vi "Get Data Replay Loop Component Properties.vi"(8 "error in (no error)":errorcluster, 11 "Item Ref in":T3 format="%.0x") -> (0 "error out":errorcluster, 2 "DataReplayLoops":T1[](array[typedef]), 3 "Item Ref out":T3 format="%.0x")   [LabVIEW 2011, in "Engine Sim System Explorer.lvlib"]
uses:
  Engine Sim System Explorer.lvlib
  <vilib>/NI Veristand/Custom Device API/Custom Device Item Ref.ctl
  TypeDefs/DataReplayLoopComp.ctl
  TypeDefs/DataReplayComp.ctl
  Shared/Engine Simulation Global.vi
  <vilib>/NI Veristand/Custom Device API/Get Item Property (I32).vi
  <vilib>/NI Veristand/Custom Device API/Get Item Property (String).vi
  Engine Simulation Shared.lvlib
  <vilib>/NI Veristand/Custom Device API/Custom Device API.lvlib
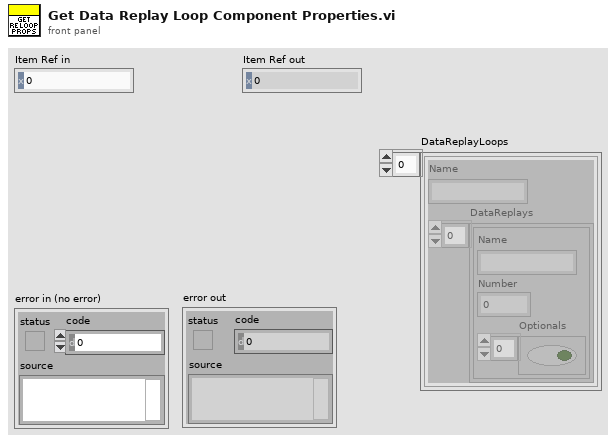
[diagram p1: front panel]
types:
  T1 = typedef "Engine Sim System Explorer.lvlib/DataReplayLoopComp.ctl" = cluster{"Name":string, "DataReplays":T2[]}
  T2 = typedef "Engine Sim System Explorer.lvlib/DataReplayComp.ctl" = cluster{"Name":string, "Number":i32, "Optionals":bool[]}
  T3 = typedef "Custom Device API.lvlib/Custom Device Item Ref.ctl" = u64
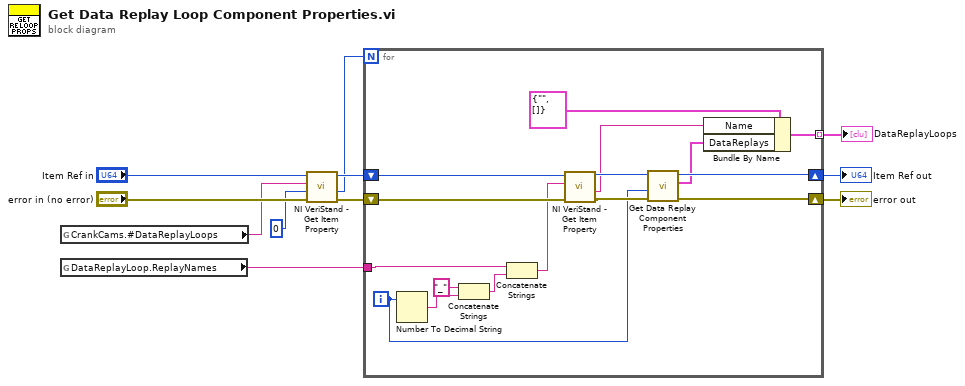
[diagram p0: block diagram]
diagram:
  n1 = global read "Engine Simulation Global.vi" "CrankCams.#DataReplayLoops"() -> (w9:string)
  n2 = global read "Engine Simulation Global.vi" "DataReplayLoop.ReplayNames"() -> (w6:string)
  n3 = call-poly <vilib>:"NI VeriStand - Get Item Property.vi"("error in (no error)"="error in (no error)", "Default Value"=0, "Property Name"=w9, "Item Ref in"="Item Ref in") -> ("error out"=w8:errorcluster, "Value"=w2:i32, "Item Ref out"=w7:T3)  [unwired: 4 in, 1 out]
  n4 = for {
    N: w2 -> [_]
    shift-right: [w17] -> w5
    shift-left: w8 -> [w24]
    shift-right: [w18] -> w4
    shift-left: w7 -> [w23]
    tunnel: w6 -> [w27]
    tunnel: [w12] -> w1 mode=indexing
    i -> [w16]
    n5 = Number To Decimal String(number=w16) -> (decimal integer string=w26:string)  [unwired: 1 in]
    n6 = Concatenate Strings("_" ("string"), w26) -> (w21:string)
    n7 = Concatenate Strings(w27, w21) -> (w22:string)
    n8 = call-poly <vilib>:"NI VeriStand - Get Item Property.vi"("error in (no error)"=w24, "Property Name"=w22, "Item Ref in"=w23) -> ("error out"=w20:errorcluster, "Value"=w14:string, "Item Ref out"=w19:T3)  [unwired: 5 in, 1 out]
    n9 = call "Get Data Replay Component Properties.vi"("error in (no error)"=w20, "ReplayLoop #"=w16, "Item Ref in"=w19) -> ("error out"=w17:errorcluster, "DataReplays"=w13:T2[], "Item Ref out"=w18:T3)  [unwired: 6 in]
    n10 = Bundle By Name(cluster=T1 {"Name"="", "DataReplays"=[]} ("DataReplayLoop"), "Name"=w14, "DataReplays"=w13) -> (w12:T1)
  }
  "error out" <- w5
  "Item Ref out" <- w4
  "DataReplayLoops" <- w1
